vi "Read Elevator Constants from Config.vi"(8 "error in (no error)":errorcluster, 11 "Settings":variant) -> (0 "error out":errorcluster, 2 "Elevator Constants":T1, 3 "Settings out":variant)   [LabVIEW 2018, in "Elevator.lvlib" / "Elevator.lvclass"]
doc: "This VI reads the elevator constants from the variant with the configuration. It returns the type def of constants"
uses:
  Elevator.lvclass
  Controls/Elevator Constants.ctl
  4aa940ad-1d57-42ab-8d63-0c1305937079.vi
  0b288b29-b09c-419b-95f0-94f636d0143a.vi
  <vilib>/Utility/error.llb/Error Cluster From Error Code.vi
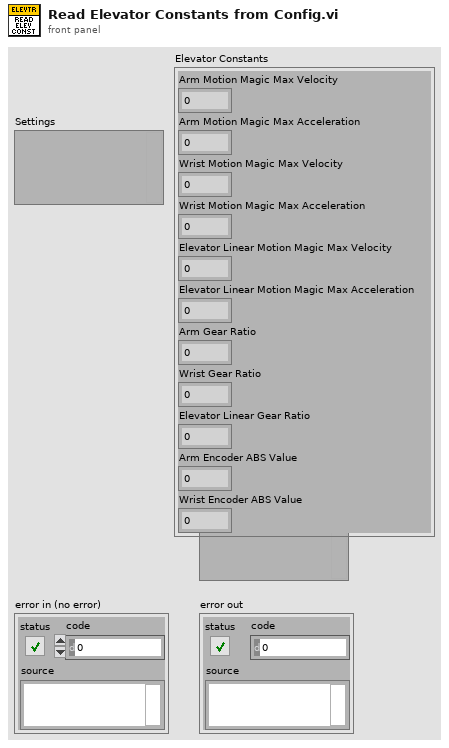
[diagram p1: front panel]
types:
  T1 = typedef "Elevator.lvlib/Elevator.lvclass/Elevator Constants.ctl" = cluster{"Arm Motion Magic Max Velocity":u32, "Arm Motion Magic Max Acceleration":u32, "Wrist Motion Magic Max Velocity":u32, "Wrist Motion Magic Max Acceleration":u32, "Elevator Linear Motion Magic Max Velocity":u32, "Elevator Linear Motion Magic Max Acceleration":u32, "Arm Gear Ratio":dbl, "Wrist Gear Ratio":dbl, "Elevator Linear Gear Ratio":dbl, "Arm Encoder ABS Value":i32, "Wrist Encoder ABS Value":i32}
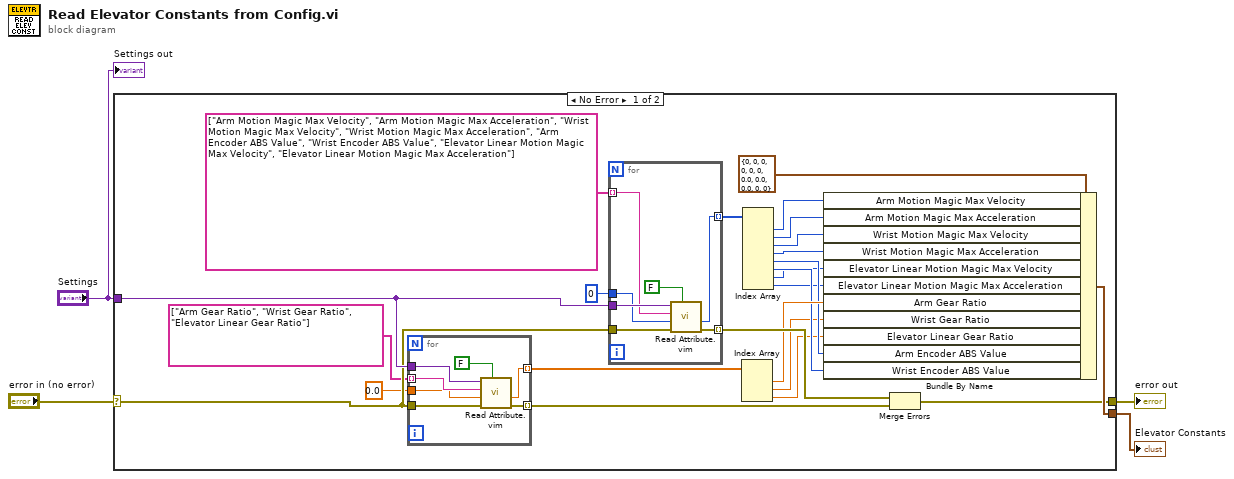
[diagram p0: block diagram]
diagram:
  n1 = case shown="No Error" "error in (no error)" {
    selector: "error in (no error)" -> [w22 w43]
    tunnel: "Settings" -> [w25 _]
    tunnel: [w24 w43] -> w3
    tunnel: [w28 _] -> w2
    frame No Error {
      n2 = for {
        tunnel: w25 -> [w42]
        tunnel: w22 -> [w41]
        tunnel: [w40] -> w26 mode=indexing
        tunnel: string[] ["Arm Gear Ratio", "Wrist Gear Ratio", "Elevator Linear Gear Ratio"] ("keys") -> [w39] mode=indexing
        tunnel: 0.0 -> [w38]
        tunnel: [w37] -> w16 mode=indexing
        n3 = call "Read Attribute.vim"("Error if not found (T)"=FALSE, "error in"=w41, "default value (data type)"=w38, "name"=w39, "variant in"=w42) -> ("error out"=w40:errorcluster, "value"=w37:dbl)  [unwired: 3 in, 2 out]
      }
      n4 = for {
        tunnel: w25 -> [w33]
        tunnel: w22 -> [w35]
        tunnel: [w34] -> w23 mode=indexing
        tunnel: string[] ["Arm Motion Magic Max Velocity", "Arm Motion Magic Max Acceleration", "Wrist Motion Magic Max Velocity", "Wrist Motion Magic Max Acceleration", "Arm Encoder ABS Value", "Wrist Encoder ABS Value", "Elevator Linear Motion Magic Max Velocity", "Elevator Linear Motion Magic Max Acceleration"] ("PID Sections to read") -> [w32] mode=indexing
        tunnel: u32 0 -> [w31]
        tunnel: [w30] -> w17 mode=indexing
        n5 = call "Read Attribute.vim"("Error if not found (T)"=FALSE, "error in"=w35, "default value (data type)"=w31, "name"=w32, "variant in"=w33) -> ("error out"=w34:errorcluster, "value"=w30:u32)  [unwired: 3 in, 2 out]
      }
      n6 = Index Array(array=w16) -> (element #1=w15:dbl, element #2=w8:dbl, element #3=w5:dbl)  [unwired: 3 in]
      n7 = Index Array(array=w17) -> (element #1=w14:u32, element #2=w13:u32, element #3=w12:u32, element #4=w11:u32, element #5=w10:u32, element #6=w9:u32, element #7=w7:u32, element #8=w6:u32)  [unwired: 8 in]
      n8 = Bundle By Name(cluster=T1 {"Arm Motion Magic Max Velocity"=0, "Arm Motion Magic Max Acceleration"=0, "Wrist Motion Magic Max Velocity"=0, "Wrist Motion Magic Max Acceleration"=0, "Elevator Linear Motion Magic Max Velocity"=0, "Elevator Linear Motion Magic Max Acceleration"=0, "Arm Gear Ratio"=0.0, "Wrist Gear Ratio"=0.0, "Elevator Linear Gear Ratio"=0.0, "Arm Encoder ABS Value"=0, "Wrist Encoder ABS Value"=0} ("Elevator Constants"), "Arm Motion Magic Max Velocity"=w14, "Arm Motion Magic Max Acceleration"=w13, "Wrist Motion Magic Max Velocity"=w12, "Wrist Motion Magic Max Acceleration"=w11, "Elevator Linear Motion Magic Max Velocity"=w7, "Elevator Linear Motion Magic Max Acceleration"=w6, "Arm Gear Ratio"=w15, "Wrist Gear Ratio"=w8, "Elevator Linear Gear Ratio"=w5, "Arm Encoder ABS Value"=w10, "Wrist Encoder ABS Value"=w9) -> (w28:T1)
      n9 = Merge Errors(w23, w26) -> (w24:errorcluster)
    }
    frame Error {
    }
  }
  "error out" <- w3
  "Elevator Constants" <- w2
  "Settings out" <- "Settings"
